vi "getCorners.vi"(8 "error in (no error)":errorcluster, 11 "StationKeeping in":refnum<class "StationKeeping.lvclass">) -> (0 "error out":errorcluster, 2 "output array":T1[](array[typedef]) {"North" format="%#_10f"; "East" format="%#_8f"}, 3 "StationKeeping out":refnum<class "StationKeeping.lvclass">)   [LabVIEW 2013, in "StationKeeping.lvclass"]
doc: "Returns the four corners of the station keeping box in no particular order\n\nAssumes the station keeping box is square\nBox can be at any arbitrary angle"
uses:
  StationKeeping.lvclass
  Data/TypeDefs/UTM Location.ctl
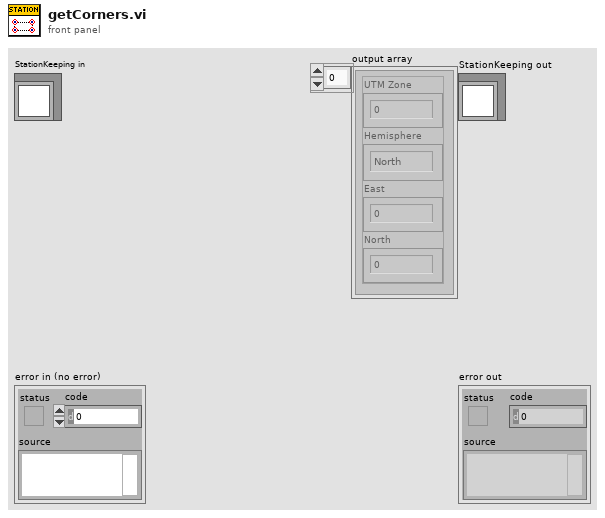
[diagram p1: front panel]
types:
  T1 = typedef "UTM Location.ctl" = cluster{"UTM Zone":dbl, "Hemisphere":enum16{"North", "South"}, "East":dbl, "North":dbl}
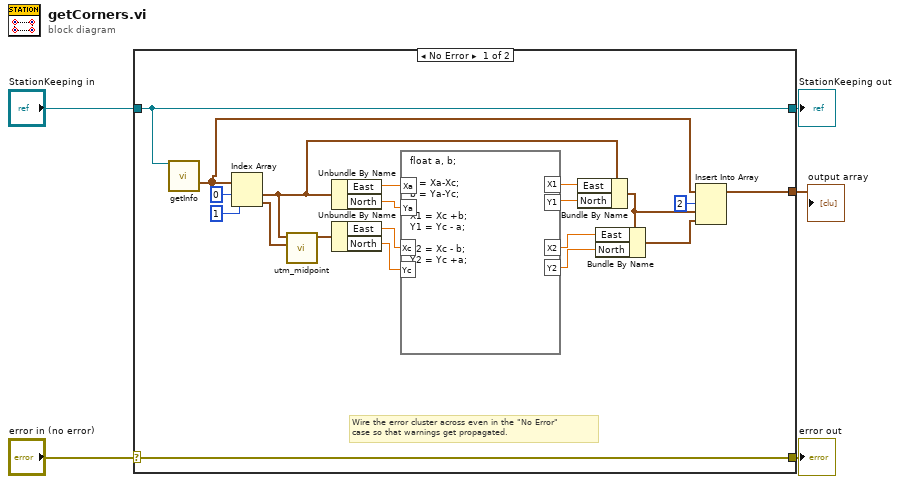
[diagram p0: block diagram]
diagram:
  n1 = case shown="No Error" "error in (no error)" {
    selector: "error in (no error)" -> [w25 w27]
    tunnel: [w25 w27] -> w4
    tunnel: [w24 w26] -> w2
    tunnel: "StationKeeping in" -> [w24 w26]
    tunnel: [w17 _] -> w1
    frame No Error {
      # "Wire the error cluster across even in the \"No Error\"\ncase so that warnings get propagated."
      n2 = call-dynamic "getInfo.vi"("GenericMission in"=w24) -> ("Points of Interest"=w21:T1[])  [unwired: 6 in, 8 out]
      n3 = Index Array(array=w21, index #1=0 ("index"), index #2=1 ("index")) -> (element #1=w7:T1, element #2=w8:T1)
      n4 = call "utm_midpoint.vi"("UTM Location 2"=w8, "UTM Location"=w7) -> ("UTM Location 3"=w6:T1)  [unwired: 7 in, 2 out]
      n5 = Unbundle By Name(w7) -> ("East"=w12:dbl, "North"=w11:dbl)
      n6 = Unbundle By Name(w6) -> ("East"=w10:dbl, "North"=w9:dbl)
      n7 = formula code="float a, b;\n\na = Xa-Xc;\nb = Ya-Yc;\n\nX1 = Xc +b;\nY1 = Yc - a;\n\nX2 = Xc - b;\nY2 = Yc +a;"("Xa"=w12, "Ya"=w11, "Xc"=w10, "Yc"=w9) -> ("X1"=w14:dbl, "Y1"=w13:dbl, "X2"=w15:dbl, "Y2"=w16:dbl)
      n8 = Bundle By Name(cluster=w7, "East"=w14, "North"=w13) -> (w20:T1)
      n9 = Bundle By Name(cluster=w20, "East"=w15, "North"=w16) -> (w19:T1)
      n10 = Insert Into Array(array=w21, index=2, new element #1=w20, new element #2=w19) -> (w17:T1[])
    }
    frame Error {
    }
  }
  "error out" <- w4
  "StationKeeping out" <- w2
  "output array" <- w1
